vi "Close All Clients.vi"(8 "error in (no error)":errorcluster, 11 "Websocket Server in":refnum<class "Websocket Server.lvclass">) -> (0 "error out":errorcluster, 2 "Timeout":bool, 3 "Websocket Server out":refnum<class "Websocket Server.lvclass">)   [LabVIEW 2020, in "Stream-Websocket.lvlib" / "Websocket Server.lvclass"]
uses:
  Websocket Server.lvclass
  Websocket Client/Websocket Client.lvclass
  C:/dev/lv20CE/relink/lv-stream/stream/Endpoint/Endpoint.lvclass
  lv-stream/stream/Endpoint/Endpoint.lvclass
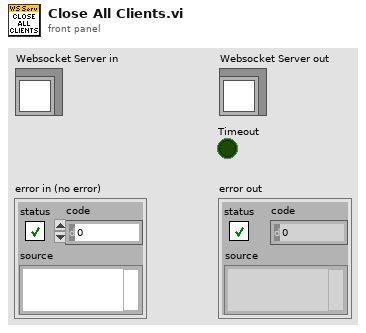
[diagram p1: front panel]
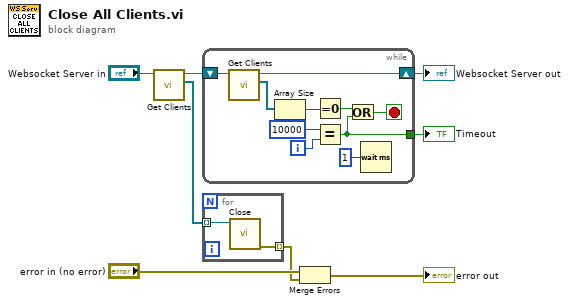
[diagram p0: block diagram]
diagram:
  n1 = call "Get Clients.vi"("Websocket Server in"="Websocket Server in") -> ("Clients"=w4:refnum<class "Websocket Client.lvclass">[], "Websocket Server out"=w3:refnum<class "Websocket Server.lvclass">)  [unwired: 8 in, 1 out]
  n2 = while {
    shift-right: [w10] -> w1
    shift-left: w3 -> [w18]
    tunnel: [w11] -> w2
    i -> [w14]
    stop <- w12 stop-if-true
    n3 = call "Get Clients.vi"("Websocket Server in"=w18) -> ("Clients"=w17:refnum<class "Websocket Client.lvclass">[], "Websocket Server out"=w10:refnum<class "Websocket Server.lvclass">)  [unwired: 8 in, 1 out]
    n4 = Array Size(array=w17) -> (size(s)=w16:i32)
    n5 = Equal To 0?(x=w16) -> (x = 0?=w13:bool)
    n6 = Equal?(x=10000, y=w14) -> (x = y?=w11:bool)
    n7 = Or(x=w13, y=w11) -> (x .or. y?=w12:bool)
    n8 = Wait (ms)(milliseconds to wait=u32 1) -> ()  [unwired: 1 out]
  }
  "Websocket Server out" <- w1
  "Timeout" <- w2
  n9 = for {
    tunnel: w4 -> [w20] mode=indexing
    tunnel: [w19] -> w5 mode=indexing
    n10 = call "Close.vi"("Endpoint in"=w20) -> ("error out"=w19:errorcluster)  [unwired: 9 in, 1 out]
  }
  n11 = Merge Errors("error in (no error)", w5) -> (→"error out":errorcluster)
